vi "PSCHN_JudgeClick.vi"(7 "Coords":T1, 8 "Error In (no error)":errorcluster, 9 "Q_Name":string, 10 "PopUp Name":string, 11 "TreeRef":refnum<vi>) -> (0 "Error Out":errorcluster)   [LabVIEW 2016]
uses:
  <vilib>/Utility/miscctls.llb/LVPoint32TypeDef.ctl
  <vilib>/Pansino Software/LabVIEW Architecture/Queue Management/PSARC_Queue Insert Element.vi
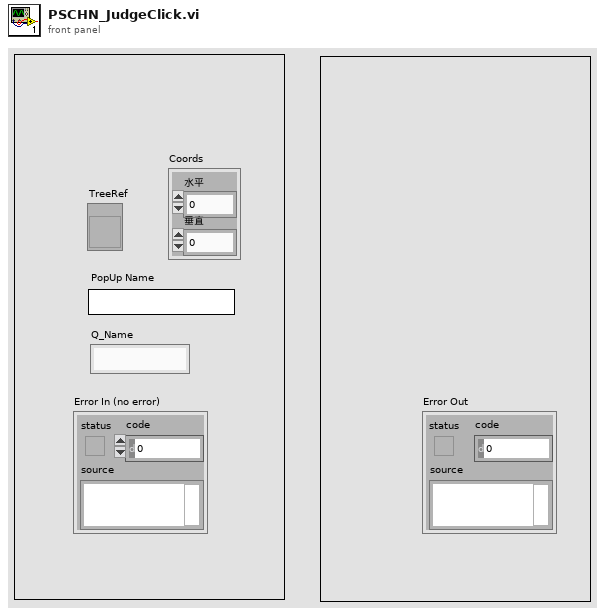
[diagram p1: front panel]
types:
  T1 = typedef "LVPoint32TypeDef.ctl" = cluster{"Horizontal":i32, "Vertical":i32}
  T2 = typedef "PSPOP_Popup Call Parameters.ctl" = cluster{"Prop Type":T3, "Initial Value":variant, "Caption Strings":string[], "Ring Strings":string[], "Cell Rect":cluster{"left":i16, "top":i16, "right":i16, "bottom":i16}, "Mouse Coords":cluster{"x":i16, "y":i16}, "Call Data":variant, "Ring Values":ext[], "Browse Options":T4, "Combo Box":cluster{"Allow Undefined Strings":bool}}
  T3 = typedef "PSPOP_Data Type.ctl" = enum16{"NO POPUP", "Unkown", "String", "Integer", "Float", "Color", "Boolean", "Ring", "Captioned String", "Captioned Integer", "Button Color", "2 Int Cluster", "4 Int Cluster", "6-Dbl Cluster", "Path", "Combox", "Time", "ShotCut String"}
  T4 = typedef "LVBrowseOptionsTypeDef.ctl" = cluster{"Prompt":string, "Match Pattern":string, "Mode":enum32{"existing file", "new file", "new or existing file", "existing dir", "new dir", "new or existing dir", "existing file (use LLBs)", "new file (use LLBs)", "new or existing file (use LLBs)", "new or existing file or directory (use LLBs)", "existing dir (use LLBs)", "new dir (use LLBs)", "new or existing dir (use LLBs)", "existing file or dir", "new file or dir", "new or existing file or dir", "existing file or dir (use LLBs)", "new file or dir (use LLBs)"}, "Start Path":path, "Pattern Label":string, "Button Text":string}
  T5 = typedef "PSPOP_Grid.Cell Info.ctl" = cluster{"Tag":string, "Row":i32, "Column":i32, "In Symbol?":bool, "In Data?":bool, "Cell String":string, "Ctl Refnum":refnum<vi>, "Prop Type":T3, "Ring Strings":string[], "Ring Values":ext[], "New Cell String":string}
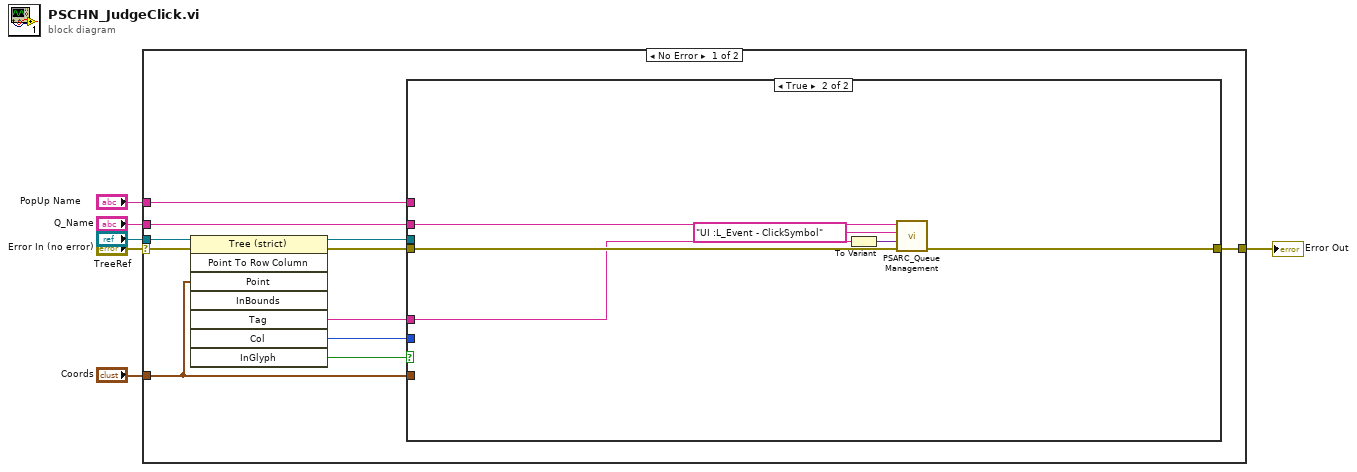
[diagram p0: block diagram]
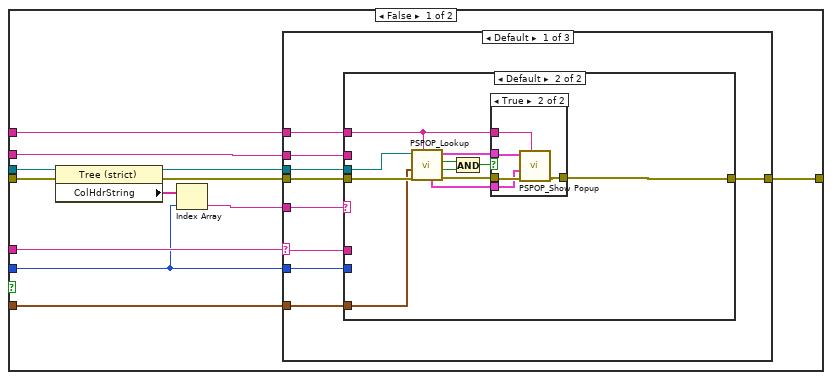
[diagram p2: hidden frame]
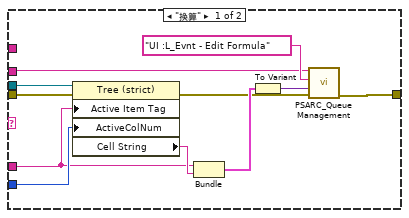
[diagram p3: hidden frame]
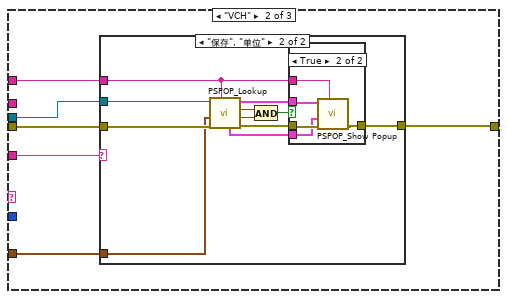
[diagram p5: hidden frame]
diagram:
  n1 = case shown="No Error" "Error In (no error)" {
    selector: "Error In (no error)" -> [w7 w98]
    tunnel: "Coords" -> [w16 _]
    tunnel: "PopUp Name" -> [w15 _]
    tunnel: "TreeRef" -> [w10 _]
    tunnel: "Q_Name" -> [w9 _]
    tunnel: [w8 w98] -> w2
    frame No Error {
      n2 = invoke class="Tree (strict)" method="Point To Row Column"(reference=w10, error in=w7, "Point"=w16) -> (reference out=w14:refnum<vi>, error out=w12:errorcluster, "Tag"=w13:string, "Col"=w17:i32, "InGlyph"=w11:bool)  [unwired: 5 in, 3 out]
      n3 = case shown="True" w11 {
        tunnel: [w28 w96] -> w8
        tunnel: w9 -> [w19 w95]
        tunnel: w12 -> [w24 w93]
        tunnel: w13 -> [w29 w92]
        tunnel: w14 -> [w25 _]
        tunnel: w15 -> [w27 _]
        tunnel: w16 -> [w26 _]
        tunnel: w17 -> [w18 _]
        frame False {
          n4 = property class="Tree (strict)"(reference=w25, error in=w24) -> (reference out=w23:refnum<vi>, error out=w21:errorcluster, "ColHdrString"=w22:string[])
          n5 = Index Array(array=w22, index=w18) -> (element=w20:string)
          n6 = case shown="Default" w29 {
            selector: w29 -> [w31 _ _]
            tunnel: w21 -> [w37 w71 w91]
            tunnel: [w38 w72 w91] -> w28
            tunnel: w23 -> [w36 w70 _]
            tunnel: w27 -> [w35 w69 _]
            tunnel: w26 -> [w34 w68 _]
            tunnel: w20 -> [w33 w67 _]
            tunnel: w18 -> [w32 _ _]
            tunnel: w19 -> [w30 _ _]
            frame Default {
              n7 = case shown="Default" w33 {
                tunnel: [w39 w54] -> w38
                tunnel: w37 -> [w43 w53]
                tunnel: w36 -> [w40 w52]
                tunnel: w35 -> [_ w51]
                tunnel: w34 -> [_ w50]
                tunnel: w32 -> [w44 _]
                tunnel: w31 -> [w42 _]
                tunnel: w30 -> [w41 _]
                frame "换算" {
                  n8 = property class="Tree (strict)"(reference=w40, error in=w43, "Active Item Tag"=w42, "ActiveColNum"=w44) -> (error out=w45:errorcluster, "Cell String"=w47:string)  [unwired: 1 out]
                  n9 = Bundle(w42, "Cell String"=w47) -> (w46:cluster{string, "Cell String":string})  [unwired: 1 in]
                  n10 = To Variant(anything=w46) -> (Variant=w48:variant)
                  n11 = call-poly <vilib>:"PSARC_Queue Management.vi"("error in (no error)"=w45, "Data"=w48, "Event"="UI :L_Evnt - Edit Formula", "Queue Name(unamed)"=w41) -> ("error out"=w39:errorcluster)  [unwired: 6 in, 1 out]
                }
                frame Default {
                  n12 = call <vilib>:"PSPOP_Lookup.vi"("Name"=w51, "error in (no error)"=w53, "Point"=w50, "Ctl Refnum"=w52) -> ("error out"=w56:errorcluster, "In Bounds?"=w60:bool, "Found"=w59:bool, "Popup Parameters"=w57:T2, "Cell Info (Call data)"=w58:T5)  [unwired: 3 in]
                  n13 = And(x=w59, y=w60) -> (x .and. y?=w55:bool)
                  n14 = case shown="True" w55 {
                    tunnel: w56 -> [w61 w65]
                    tunnel: w57 -> [_ w66]
                    tunnel: [w61 w64] -> w54
                    tunnel: w58 -> [_ w63]
                    tunnel: w51 -> [_ w62]
                    frame False {
                    }
                    frame True {
                      n15 = call <vilib>:"PSPOP_Show Popup.vi"("Name"=w62, "error in (no error)"=w65, "Call Data (ignore if empty)"=w63, "Popup Parameters"=w66) -> ("error out"=w64:errorcluster)  [unwired: 7 in]
                    }
                  }
                }
              }
            }
            frame "VCH" {
              n16 = case shown="\"保存\", \"单位\"" w67 {
                tunnel: [w73 w78] -> w72
                tunnel: w71 -> [w73 w77]
                tunnel: w70 -> [_ w76]
                tunnel: w69 -> [_ w75]
                tunnel: w68 -> [_ w74]
                frame Default {
                }
                frame "保存", "单位" {
                  n17 = call <vilib>:"PSPOP_Lookup.vi"("Name"=w75, "error in (no error)"=w77, "Point"=w74, "Ctl Refnum"=w76) -> ("error out"=w80:errorcluster, "In Bounds?"=w84:bool, "Found"=w83:bool, "Popup Parameters"=w81:T2, "Cell Info (Call data)"=w82:T5)  [unwired: 3 in]
                  n18 = And(x=w83, y=w84) -> (x .and. y?=w79:bool)
                  n19 = case shown="True" w79 {
                    tunnel: w80 -> [w85 w89]
                    tunnel: w81 -> [_ w90]
                    tunnel: [w85 w88] -> w78
                    tunnel: w82 -> [_ w87]
                    tunnel: w75 -> [_ w86]
                    frame False {
                    }
                    frame True {
                      n20 = call <vilib>:"PSPOP_Show Popup.vi"("Name"=w86, "error in (no error)"=w89, "Call Data (ignore if empty)"=w87, "Popup Parameters"=w90) -> ("error out"=w88:errorcluster)  [unwired: 7 in]
                    }
                  }
                }
              }
            }
            frame "" {
            }
          }
        }
        frame True {
          n21 = To Variant(anything=w92) -> (Variant=w94:variant)
          n22 = call-poly <vilib>:"PSARC_Queue Management.vi"("error in (no error)"=w93, "Data"=w94, "Event"="UI :L_Event - ClickSymbol", "Queue Name(unamed)"=w95) -> ("error out"=w96:errorcluster)  [unwired: 6 in, 1 out]
        }
      }
    }
    frame Error {
    }
  }
  "Error Out" <- w2
